vi "h5_config_flatten.vi"(10 "scan_config":T1={"v0 name"="radiant (nm)", "v0 num"=808, "v1 name"="none", "v1 num"=808, "scan_values"=[], "num rows"=808, "measurement"=0, "v0_config"={"hardware"=enum."radiant (nm)", "options"="", "repeats"=4, "loops"=1, "VISA"="COM9", "override_VISA"=TRUE}, "v1_config"={"hardware"=enum."radiant (nm)", "options"="", "repeats"=4, "loops"=1, "VISA"="COM9", "override_VISA"=TRUE}, "scope_config"={"VISA"="lecroy", "channels"=[enum."Channel 1"], "timeout (ms)"=100000, "max_points"=2500, "averages"=50, "noise filter"=enum."None"}} {"scope_config"."averages" min=1; "scope_config"."max_points" items=["50"=50, "100"=100, "250"=250, "500"=500, "1000"=1000, "2500"=2500, "5K"=5000, "10K"=10000, "25K"=25000, "50K"=50000, "100K"=100000, "250K"=250000, "500K"=500000, "1M"=1000000, "2M"=2000000, "2.5M"=2500000, "5M"=5000000, "10M"=10000000, "25M"=25000000, "50M"=50000000, "100M"=100000000]; "v1_config"."loops" min=1; "v1_config"."repeats" min=1; "v0_config"."loops" min=1; "v0_config"."repeats" min=1}) -> (1 "Values out":variant[](array[variant]), 2 "Names out":string[](array[string]))   [LabVIEW 2017, in "tools.lvlib"]
uses:
  core/scan_config.ctl
  core/var_config.ctl
  ctrl/var_list.ctl
  hardware/lecroy/scope_config.ctl
  <vilib>/Utility/VariantDataType/GetClusterInfo.vi
  <vilib>/Utility/VariantDataType/GetTypeInfo.vi
  <vilib>/UPVI/lvhdf5/attribute.llb/Cluster to Attribute Array.xnode
  tools.lvlib
  <vilib>/Utility/VariantDataType/VariantType.lvlib
  hardware/lecroy/lecroy.lvlib
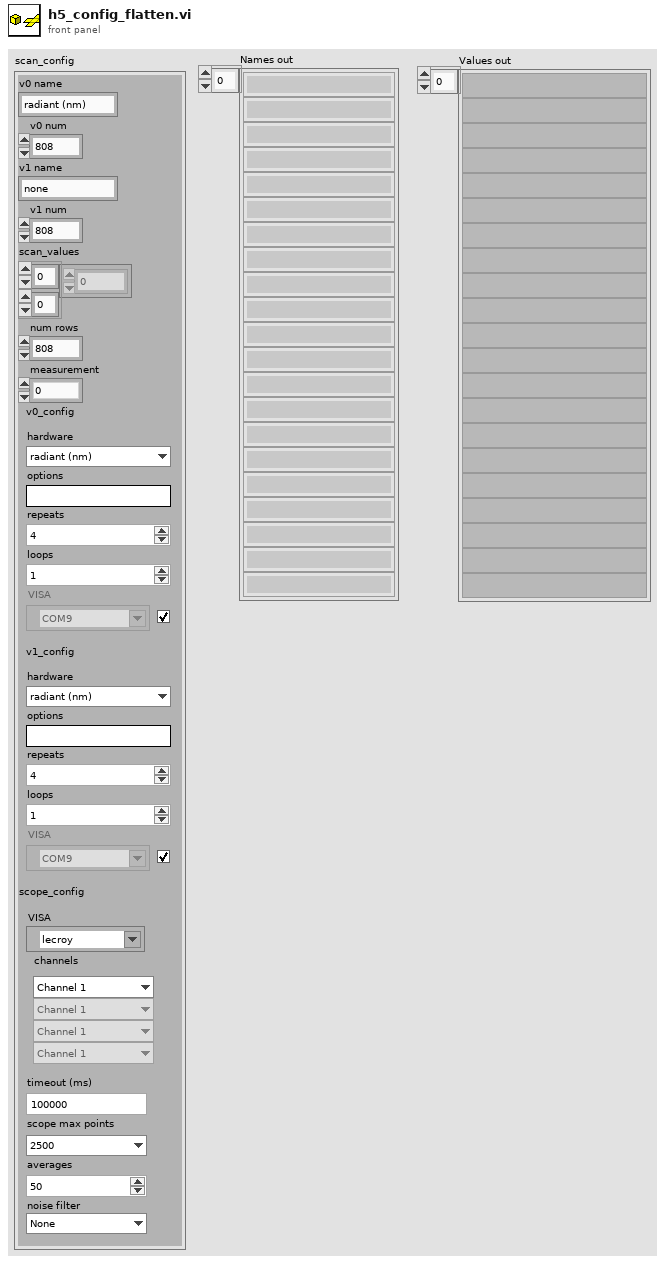
[diagram p1: front panel]
types:
  T1 = typedef "tools.lvlib/scan_config.ctl" = cluster{"v0 name":string, "v0 num":i32, "v1 name":string, "v1 num":i32, "scan_values":dbl[][], "num rows":i32, "measurement":i32, "v0_config":T2, "v1_config":T2, "scope_config":T4}
  T2 = typedef "tools.lvlib/var_config.ctl" = cluster{"hardware":T3, "options":string, "repeats":i32, "loops":i32, "VISA":refnum<visa-resource-name>, "override_VISA":bool}
  T3 = typedef "var_list.ctl" = enum16{"none", "AO voltage (V)", "delay (s)", "generic", "microwaves (GHz)", "radiant (nm)", "radiant thg (nm)", "sirah (nm)", "sirah_shg (nm)", "tenma voltage (V)", "wait (s)", "wf_freq (Hz)", "wf_amp (V)", "wf_amp_multi (V)", "wf_offset (V)", "wf_low_level (V)", "wf_high_level (V)", "wf_period (s)", "wf_pulse_width (s)", "wf_sample_rate (Sa/s)", "wf_multi_amp", "wf_multi_freq", "wf_arb_4chan", "WS7 setpoint (nm)"}
  T4 = typedef "lecroy.lvlib/scope_config.ctl" = cluster{"VISA":refnum<visa-resource-name>, "channels":enum16{"Channel 1", "Channel 2", "Channel 3", "Channel 4"}[], "timeout (ms)":u32, "max_points":i32, "averages":i32, "noise filter":enum16{"None", "+0.5 bit", "+1 bit", "+1.5 bits", "+2 bits", "+2.5 bits", "+3 bits"}}
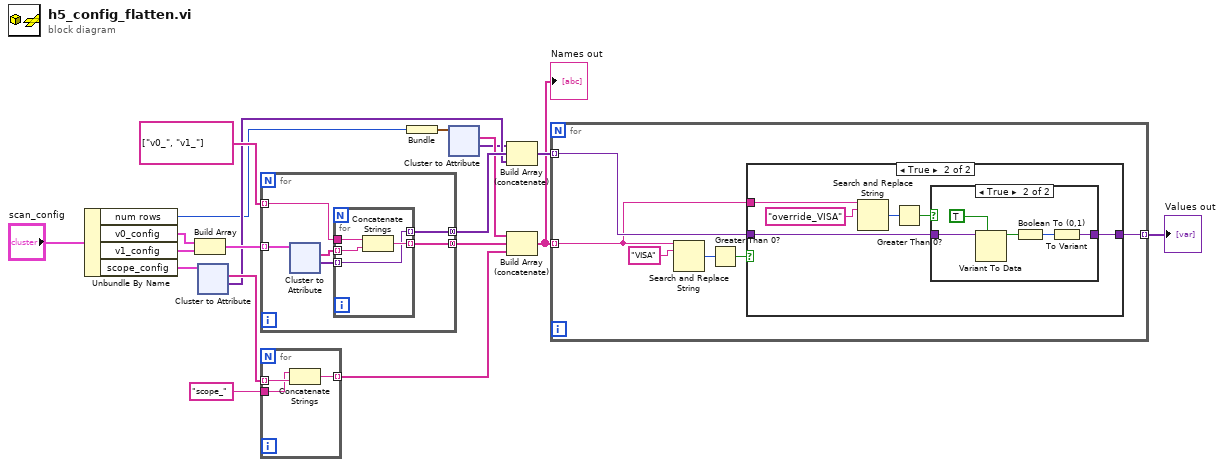
[diagram p0: block diagram]
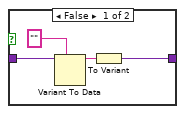
[diagram p3: hidden frame]
diagram:
  n1 = Unbundle By Name("scan_config") -> ("num rows"=w7:i32, "v0_config"=w17:T2, "v1_config"=w16:T2, "scope_config"=w14:T4)
  n2 = Build Array(w17, w16) -> (w15:T2[])
  n3 = xnode "Cluster to Attribute"("Cluster"=w14) -> ("Names out"=w12:string[], "Values out"=w8:variant[])  [unwired: 5 in, 1 out]
  n4 = for {
    tunnel: string[] ["v0_", "v1_"] ("Array") -> [w23] mode=indexing
    tunnel: w15 -> [w25] mode=indexing
    tunnel: [w20] -> w9 mode=concatenating
    tunnel: [w22] -> w11 mode=concatenating
    n5 = xnode "Cluster to Attribute"("Cluster"=w25) -> ("Names out"=w24:string[], "Values out"=w21:variant[])  [unwired: 5 in, 1 out]
    n6 = for {
      tunnel: w24 -> [w29] mode=indexing
      tunnel: w23 -> [w28]
      tunnel: [w27] -> w22 mode=indexing
      tunnel: w21 -> [w26] mode=indexing
      tunnel: [w26] -> w20 mode=indexing
      n7 = Concatenate Strings(w28, w29) -> (w27:string)
    }
  }
  n8 = for {
    tunnel: w12 -> [w117] mode=indexing
    tunnel: "scope_" -> [w116]
    tunnel: [w115] -> w10 mode=indexing
    n9 = Concatenate Strings(w116, w117) -> (w115:string)
  }
  n10 = Bundle("num rows"=w7) -> (w6:cluster{"num rows":i32})  [unwired: 1 in]
  n11 = xnode "Cluster to Attribute"("Cluster"=w6) -> ("Names out"=w5:string[], "Values out"=w4:variant[])  [unwired: 5 in, 1 out]
  n12 = Build Array (concatenate)(w4, w9, w8) -> (w3:variant[])
  n13 = Build Array (concatenate)(w5, w11, w10) -> (w1:string[])
  "Names out" <- w1
  n14 = for {
    tunnel: w1 -> [w118] mode=indexing
    tunnel: w3 -> [w120] mode=indexing
    tunnel: [w119] -> w2 mode=indexing
    n15 = Search and Replace String(input string=w118, search string="VISA") -> (number of replacements=w122:i32)  [unwired: 6 in, 3 out]
    n16 = Greater Than 0?(x=w122) -> (x > 0?=w121:bool)
    n17 = case shown="True" w121 {
      tunnel: w120 -> [w124 w129]
      tunnel: [w124 w130] -> w119
      tunnel: w118 -> [_ w127]
      frame False {
      }
      frame True {
        n18 = Search and Replace String(input string=w127, search string="override_VISA") -> (number of replacements=w126:i32)  [unwired: 6 in, 3 out]
        n19 = Greater Than 0?(x=w126) -> (x > 0?=w125:bool)
        n20 = case shown="True" w125 {
          tunnel: [w131 w139] -> w130
          tunnel: w129 -> [w132 w138]
          frame False {
            n21 = Variant To Data(type="", Variant=w132) -> (data=w134:string)  [unwired: 1 in, 1 out]
            n22 = To Variant(anything=w134) -> (Variant=w131:variant)
          }
          frame True {
            n23 = Variant To Data(type=TRUE, Variant=w138) -> (data=w136:bool)  [unwired: 1 in, 1 out]
            n24 = Boolean To (0,1)(Boolean=w136) -> (0, 1=w135:i16)
            n25 = To Variant(anything=w135) -> (Variant=w139:variant)
          }
        }
      }
    }
  }
  "Values out" <- w2
